vi "FGV-Erweiterte Bedienung.vi"(6 "Aktion":T1, 8 "Chart wechsel":bool, 11 "N2 zu PNS":bool) -> (0 "Chart wechsel":bool, 3 "N2 zu PNS":bool)   [LabVIEW 2020, in "Funktionstasten.lvlib"]
doc: "Führt die durch den Enum \"Aktion\" geforderte Aktion aus, indem über eine Referenz auf den Cluster \"Funktionstasten\" die Beschriftungen und Tastenfarben manipuliert werden. Der Eingang \"Funktionstasten\" ist neben der Referenz notwendig, um bei einer Ereignis-gesteuerten Tastenreaktion eine gedrückte Taste zui erkennen, die Latch-Verhalten hat.\n\nDie funktionale globale Variable (FGV) speichert den aktuellen Zustand der Tasten und des aktuellen Fehlerstatus. Die FGV kann von Sub-VIs und fremden VIs aufgerufen werden. Außer dem Eingang \"Aktion\" sind alle Eingänge sind nur \"empfohlen\" und nicht immer \"erforderlich\", -abhängig von der Aktion:\n\nInitialisieren:\nSpeichert eine Referenz auf den Cluster\"Funktionstasten\" und macht alle Tasten vorläufig nicht anwählbar. Erst nach dem vollständigen Hochlauf sollten die Tasten durch die Aktion \"Zustand setzen\" in einem definierten Zustand aktiviert werden. Dabei werden die Beschriftungen der Tasten vom Enum \"Zustand\" übernommen und gespeichert.\nNur Eingang \"Referenz\" erforderlich.\n\nZustand setzen:\nÄndert den Tastenzustand programmgesteuert auf den am Eingang \"Zustand\" anliegenden Wert.\nNur Eingang \"Zustand\" erforderlich.\n\nTaste gedrückt:\nMarkiert die gedrückte Taste entsprechend dem gespeicherten Fehlerzustand und liefert die ausgewählte Funktion zur Steuerung eines Zustandsautomaten.\nNur Eingang \"Funktionstasten\" erforderlich.\n\nFehler speichern:\nÜbernimmt den Eingang \"Fehler\" und speichert ihn als \"Fehler steht an\".\nNur Eingang \"Fehler\" erforderlich.\n\nZustand lesen:\nLiefert die durch den letzten Tastendruck ausgewählte, gespeicherte Funktion und den Fehlerstatus.\nKeine Eingänge notwendig.\n\nManuell:\nAktiviert den Bedienerzugriff auf die Tasten für Handbetrieb.\nKeine Eingänge notwendig.\n\nRemote:\nDie Tasten sind nur mehr über die Aktion \"Zustand setzen\" anwählbar, die aktuelle Taste und der Fehlerzustand werden aber angezeigt.\nKeine Eingänge notwendig."
uses:
  Funktionstasten.lvlib
  FGV Erweiterte Bedienung Aktion.ctl
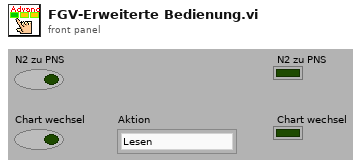
[diagram p1: front panel]
types:
  T1 = typedef "Funktionstasten.lvlib/FGV Erweiterte Bedienung Aktion.ctl" = enum16{"Lesen", "Initialisieren", "N2 zu PNS", "Chart wechsel"}
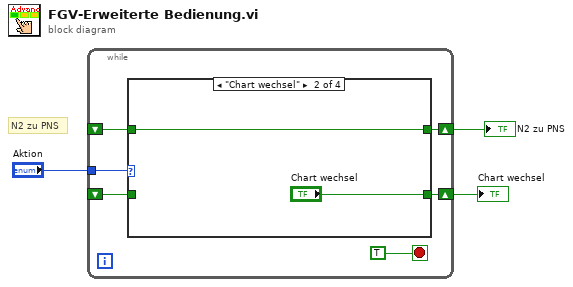
[diagram p0: block diagram]
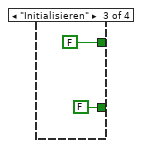
[diagram p3: hidden frame]
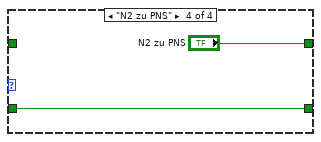
[diagram p4: hidden frame]
diagram:
  # "N2 zu PNS"
  n1 = while {
    shift-right: [w8] -> w3
    shift-left: _ -> [w7]
    tunnel: "Aktion" -> [w6]
    shift-right: [w5] -> w1
    shift-left: _ -> [w4]
    stop <- TRUE stop-if-true
    n2 = case shown="\"Chart wechsel\"" w6 {
      tunnel: [w11 w13 FALSE "N2 zu PNS"] -> w8
      tunnel: w7 -> [w11 w13 _ _]
      tunnel: [w10 "Chart wechsel" FALSE ("zu PNS Chart") w16] -> w5
      tunnel: w4 -> [w10 _ _ w16]
      frame "Lesen", Default {
      }
      frame "Chart wechsel" {
      }
      frame "Initialisieren" {
      }
      frame "N2 zu PNS" {
      }
    }
  }
  "N2 zu PNS" <- w3
  "Chart wechsel" <- w1
